vi "Routine.Export.vi"(8 "error in (no error)":errorcluster, 11 "Item Ref in":T1 format="%.0x") -> (0 "error out":errorcluster, 2 "Routine":T2 {"Stop Parameters"."Response"."Byte Order" items=["Little Endian", "Big Endian"]; "Stop Parameters"."Response"."Data Type" items=["Signed", "Unsigned", "IEEE Float"]; "Stop Parameters"."Cmd"."Byte Order" items=["Little Endian", "Big Endian"]; "Stop Parameters"."Cmd"."Data Type" items=["Signed", "Unsigned", "IEEE Float"]; "Request Parameters"."Response"."Byte Order" items=["Little Endian", "Big Endian"]; "Request Parameters"."Response"."Data Type" items=["Signed", "Unsigned", "IEEE Float"]; "Request Parameters"."Cmd"."Byte Order" items=["Little Endian", "Big Endian"]; "Request Parameters"."Cmd"."Data Type" items=["Signed", "Unsigned", "IEEE Float"]; "Start Parameters"."Response"."Byte Order" items=["Little Endian", "Big Endian"]; "Start Parameters"."Response"."Data Type" items=["Signed", "Unsigned", "IEEE Float"]; "Start Parameters"."Cmd"."Byte Order" items=["Little Endian", "Big Endian"]; "Start Parameters"."Cmd"."Data Type" items=["Signed", "Unsigned", "IEEE Float"]}, 3 "Section Ref out":T1 format="%.0x")   [LabVIEW 2015, in "Diagnostics Addon System Explorer.lvlib"]
uses:
  Diagnostics Addon System Explorer.lvlib
  <vilib>/NI Veristand/Custom Device API/Custom Device Item Ref.ctl
  Types/Routine.Export.ctl
  Types/CmdResp.Export.ctl
  Shared/Types/Signal.ctl
  Types/FG.Action.ctl
  Signals.Get.vi
  Type.FG.vi
  Signal.FG.vi
  <vilib>/NI Veristand/Custom Device API/NI VeriStand - Get Item Property.vi
  <vilib>/NI Veristand/Custom Device API/Get Item Property (U32).vi
  <vilib>/NI Veristand/Custom Device API/NI VeriStand - Set Item Property.vi
  <vilib>/NI Veristand/Custom Device API/Set Item Property (U32).vi
  Shared/SubVIs/Constants.vi
  <vilib>/NI Veristand/Custom Device API/NI VeriStand - Get Custom Device Channel Data.vi
  <vilib>/NI Veristand/Custom Device API/Get Item Property (String).vi
  <vilib>/NI Veristand/Custom Device API/Get Item Property (Double).vi
  <vilib>/NI Veristand/Custom Device API/Set Item Property (String).vi
  <vilib>/NI Veristand/Custom Device API/Set Item Property (Double).vi
  <vilib>/NI Veristand/Custom Device API/NI VeriStand - Get Item Children.vi
  <vilib>/NI Veristand/Custom Device Tools/Custom Device Utility Library/NI VeriStand - Search for Item by GUID.vi
  Shared/Diagnostics Addon Shared.lvlib
  <vilib>/NI Veristand/Custom Device API/Custom Device API.lvlib
  <vilib>/NI Veristand/Custom Device Tools/Custom Device Utility Library/Custom Device Utility Library.lvlib
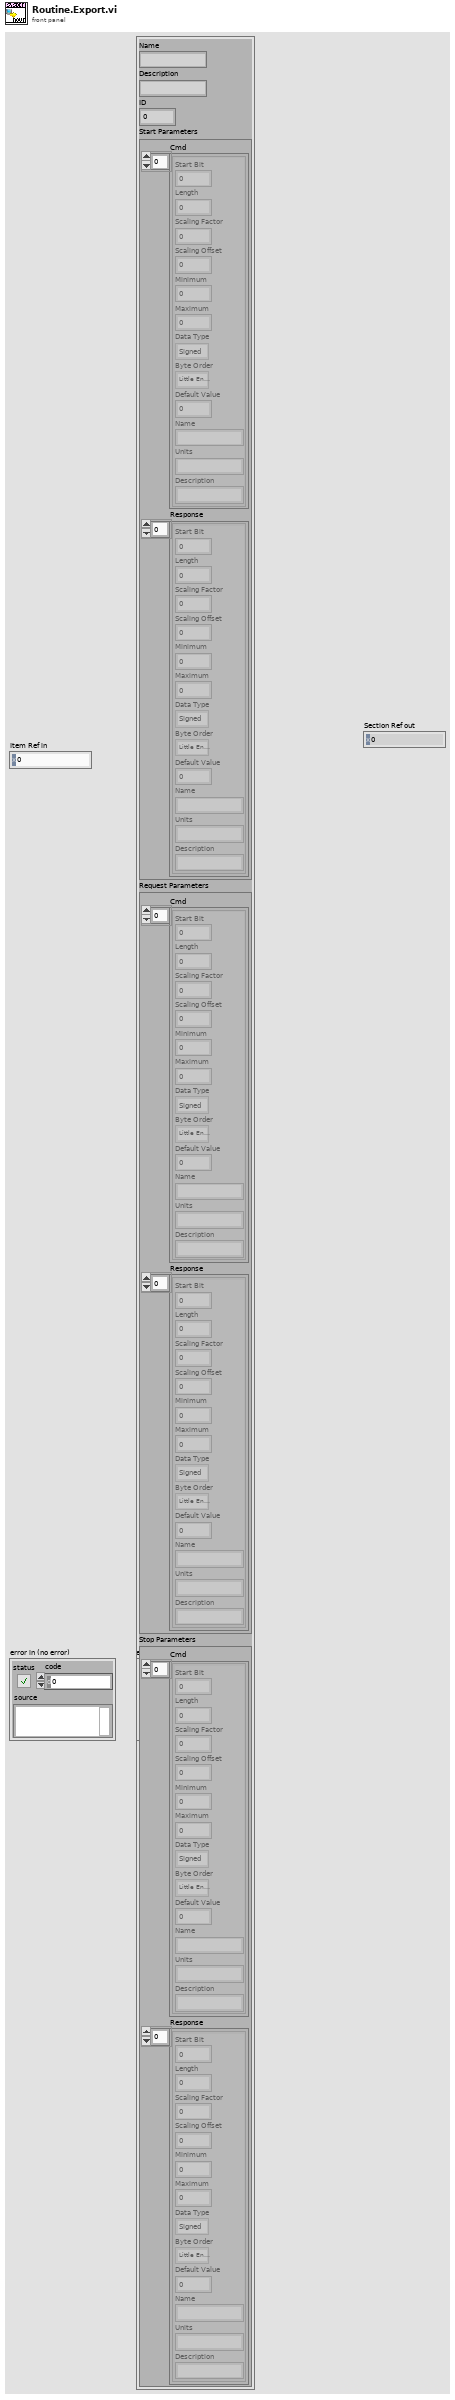
[diagram p1: front panel]
types:
  T1 = typedef "Custom Device API.lvlib/Custom Device Item Ref.ctl" = u64
  T2 = typedef "Diagnostics Addon System Explorer.lvlib/Routine.Export.ctl" = cluster{"Name":string, "Description":string, "ID":u16, "Start Parameters":T3, "Request Parameters":T3, "Stop Parameters":T3}
  T3 = typedef "Diagnostics Addon System Explorer.lvlib/CmdResp.Export.ctl" = cluster{"Cmd":T4[], "Response":T4[]}
  T4 = typedef "Diagnostics Addon Shared.lvlib/Signal.ctl" = cluster{"Start Bit":u32, "Length":u32, "Scaling Factor":dbl, "Scaling Offset":dbl, "Minimum":dbl, "Maximum":dbl, "Data Type":u32, "Byte Order":u32, "Default Value":dbl, "Name":string, "Units":string, "Description":string}
  T5 = typedef "Diagnostics Addon System Explorer.lvlib/FG.Action.ctl" = enum16{"Get", "Set"}
  T6 = typedef "Custom Device API.lvlib/Custom Device Item Info.ctl" = cluster{"Name":string, "Is Channel":bool, "GUID":string, "Is Waveform":bool}
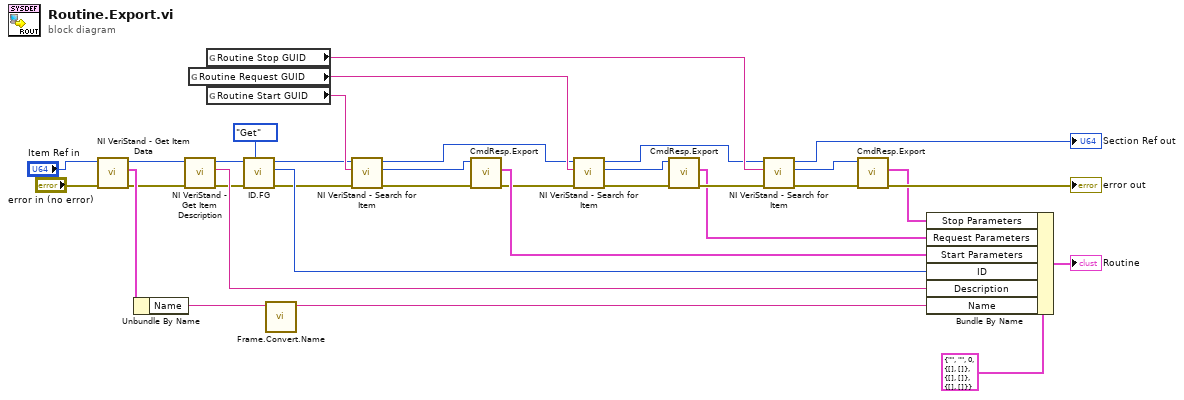
[diagram p0: block diagram]
diagram:
  n1 = call <vilib>:"NI VeriStand - Get Item Data.vi"("error in (no error)"="error in (no error)", "Item Ref in"="Item Ref in") -> ("error out"=w33:errorcluster, "Item Info"=w34:T6, "Item Ref out"=w31:T1)  [unwired: 6 in, 1 out]
  n2 = Unbundle By Name(w34) -> ("Name"=w2:string)
  n3 = call <vilib>:"NI VeriStand - Get Item Description.vi"("error in (no error)"=w33, "Item Ref in"=w31) -> ("error out"=w26:errorcluster, "Description"=w28:string, "Item Ref out"=w27:T1)  [unwired: 6 in, 1 out]
  n4 = global read "Constants.vi" "Routine Request GUID"() -> (w13:string)
  n5 = global read "Constants.vi" "Routine Stop GUID"() -> (w12:string)
  n6 = global read "Constants.vi" "Routine Start GUID"() -> (w14:string)
  n7 = call "ID.FG.vi"("Action"=FG.Action."Get", "error in (no error)"=w26, "Device Item Ref in"=w27) -> ("error out"=w24:errorcluster, "ID"=w29:u32, "Device Item Ref out"=w9:T1)  [unwired: 6 in]
  n8 = call "Frame.Convert.Name.vi"("VS Frame Name"=w2) -> ("Frame Name"=w1:string)  [unwired: 9 in, 1 out]
  n9 = call-poly <vilib>:"NI VeriStand - Search for Item.vi"("error in"=w24, "Item GUID"=w14, "Section Ref in"=w9) -> ("error out"=w17:errorcluster, "Item Ref"=w7:T1, "Section Ref out"=w8:T1)  [unwired: 5 in, 1 out]
  n10 = call "CmdResp.Export.vi"("error in (no error)"=w17, "Device Item Ref in"=w7) -> ("error out"=w20:errorcluster, "Signals"=w22:T3)  [unwired: 7 in, 1 out]
  n11 = call-poly <vilib>:"NI VeriStand - Search for Item.vi"("error in"=w20, "Item GUID"=w13, "Section Ref in"=w8) -> ("error out"=w16:errorcluster, "Item Ref"=w10:T1, "Section Ref out"=w11:T1)  [unwired: 5 in, 1 out]
  n12 = call "CmdResp.Export.vi"("error in (no error)"=w16, "Device Item Ref in"=w10) -> ("error out"=w19:errorcluster, "Signals"=w4:T3)  [unwired: 7 in, 1 out]
  n13 = call-poly <vilib>:"NI VeriStand - Search for Item.vi"("error in"=w19, "Item GUID"=w12, "Section Ref in"=w11) -> ("error out"=w15:errorcluster, "Item Ref"=w6:T1, "Section Ref out"=→"Section Ref out":T1)  [unwired: 5 in, 1 out]
  n14 = call "CmdResp.Export.vi"("error in (no error)"=w15, "Device Item Ref in"=w6) -> ("error out"=→"error out":errorcluster, "Signals"=w3:T3)  [unwired: 7 in, 1 out]
  n15 = Bundle By Name(cluster=T2 {"Name"="", "Description"="", "ID"=0, "Start Parameters"={"Cmd"=[], "Response"=[]}, "Request Parameters"={"Cmd"=[], "Response"=[]}, "Stop Parameters"={"Cmd"=[], "Response"=[]}} ("Routine"), "Stop Parameters"=w3, "Request Parameters"=w4, "Start Parameters"=w22, "ID"=w29, "Description"=w28, "Name"=w1) -> (→"Routine":T2)
